vi "DMM Read Frequery(Voltage).vi"() -> ()   [LabVIEW 2011]
uses:
  <instrlib>/DMM4/DMM4.lvlib
panel:
  out "error out":errorcluster
  out "Measure Value":string
  in  "Stop":bool
  out "Boolean":bool
  in  "Detector Rate":u16(ring) items=["SLOW", "MID", "FAST"]
  in  "Manual Range":dbl format="%#.9e"
  in  "Enable Auto Range":bool=TRUE
  out "ID Return String":string
  in  "Configure RS232 Baud Rate":u32(ring)=115200 items=["9600"=9600, "19200"=19200, "38400"=38400, "57600"=57600, "115200"=115200]
  in  "VISA resource name":refnum<visa-resource-name>
  # "DMM Read Frequery(Voltage)"
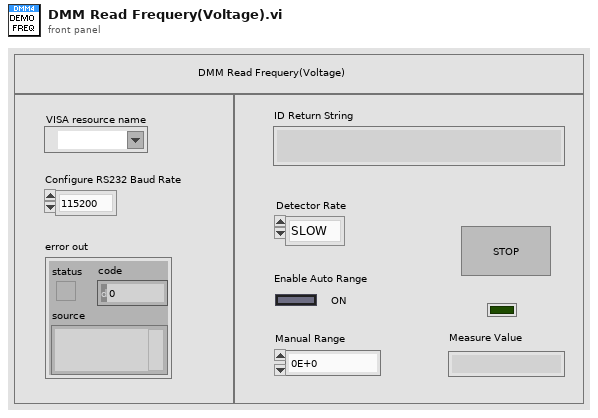
[diagram p1: front panel]
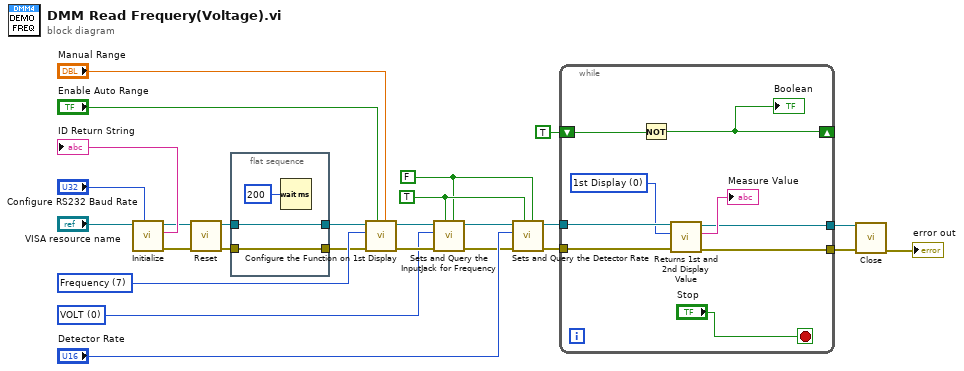
[diagram p0: block diagram]
diagram:
  w1 = u8 0 items=["VOLT", "500mA", "10A"] ("Input Jack")
  w2 = FALSE ("Enable to Query")
  w3 = TRUE ("Enable to Sets")
  w23 = u8 7 items=["DC Voltage", "AC Voltage", "DC+AC Voltage", "DC Current", "AC Current", "DC+AC Current", "2-Wire Resistance", "Frequency", "Period", "Continuity", "Diode", "Temperature", "Capacitance"] ("Function")
  n1 = call <instrlib>:"Initialize.vi"("Configure RS232 Baud Rate"="Configure RS232 Baud Rate", "VISA resource name"="VISA resource name") -> ("error out"=w13:errorcluster, "ID Return String"=→"ID Return String":string, "VISA resource name out"=w14:refnum<visa-resource-name>)  [unwired: 6 in, 1 out]
  n2 = call <instrlib>:"Reset.vi"("error in (no error)"=w13, "VISA resource name"=w14) -> ("error out"=w9:errorcluster, "VISA resource name out"=w11:refnum<visa-resource-name>)  [unwired: 8 in]
  n3 = flat-sequence {
    tunnel: w11 -> [w29]
    tunnel: [w29] -> w10
    tunnel: w9 -> [w28]
    tunnel: [w28] -> w8
    frame #0 {
      n4 = Wait (ms)(milliseconds to wait=u32 200) -> ()  [unwired: 1 out]
    }
  }
  n5 = call <instrlib>:"Configure the Function on 1st Display .vi"("Manual Range"="Manual Range", "Enable Auto Range"="Enable Auto Range", "error in"=w8, "Function"=w23, "VISA resource name"=w10) -> ("error out"=w5:errorcluster, "VISA resource name out"=w7:refnum<visa-resource-name>)  [unwired: 5 in]
  n6 = call <instrlib>:"Sets and Query the InputJack for Frequency.vi"("Enable to Query"=w2, "Enable to Sets"=w3, "error in"=w5, "Input Jack"=w1, "VISA resource name"=w7) -> ("error out"=w4:errorcluster, "VISA resource name out"=w6:refnum<visa-resource-name>)  [unwired: 4 in, 1 out]
  n7 = call <instrlib>:"Sets and Query the Detector Rate.vi"("Enable to Query"=w2, "Enable to Sets"=w3, "error in"=w4, "Detector Rate"="Detector Rate", "VISA resource name"=w6) -> ("error out"=w18:errorcluster, "VISA resource name out"=w19:refnum<visa-resource-name>)  [unwired: 4 in, 1 out]
  n8 = while {
    tunnel: w19 -> [w38]
    tunnel: w18 -> [w37]
    tunnel: [w33] -> w17
    tunnel: [w32] -> w16
    shift-right: [w30] -> _
    shift-left: TRUE -> [w31]
    stop <- "Stop" stop-if-true
    w36 = u16 0 items=["1st Display", "2nd Display", "1st & 2nd Display"] ("Sets to Display")
    n9 = Not(x=w31) -> (.not. x?=w30:bool)
    "Boolean" <- w30
    n10 = call <instrlib>:"Returns 1st and 2nd Display Value.vi"("error in"=w37, "Sets to Display"=w36, "VISA resource name"=w38) -> ("error out"=w32:errorcluster, "Return the Value"=→"Measure Value":string, "VISA resource name out"=w33:refnum<visa-resource-name>)  [unwired: 6 in]
  }
  n11 = call <instrlib>:"Close.vi"("error in (no error)"=w16, "VISA resource name"=w17) -> ("error out"=→"error out":errorcluster)  [unwired: 9 in]
